vi "Indicators (SubVI).vi"(8 "read buffer":string) -> (9 "h5":dbl, 10 "zone 3":dbl, 11 "h6":dbl caption="h4", 12 "h1":dbl, 13 "h4":dbl, 14 "inlet air":dbl, 15 "h3":dbl, 16 "t1":dbl, 17 "h2":dbl, 18 "t2":dbl, 19 "t5":dbl, 20 "zone 1":dbl, 21 "t6":dbl, 22 "outlet":dbl, 23 "t3":dbl, 24 "zone 2":dbl, 25 "t4":dbl, 26 "main return":dbl)   [LabVIEW 2019]
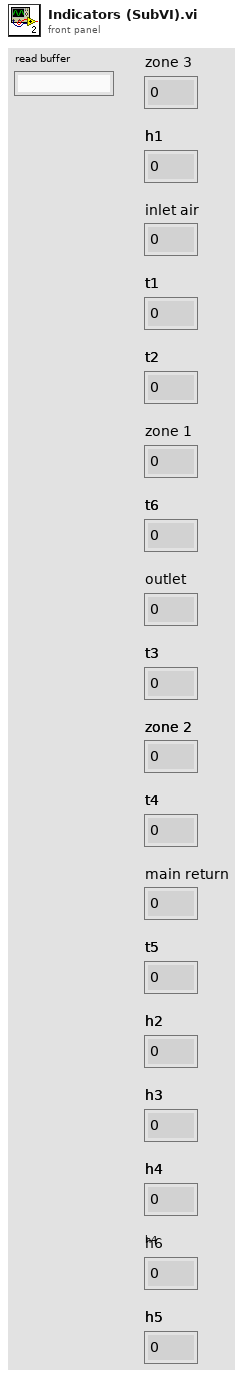
[diagram p1: front panel]
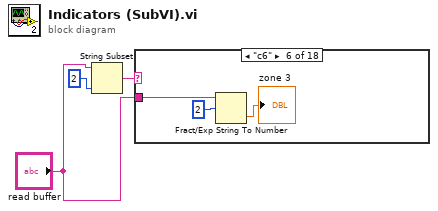
[diagram p0: block diagram]
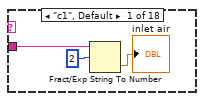
[diagram p2: hidden frame]
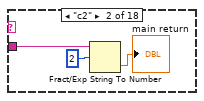
[diagram p3: hidden frame]
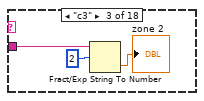
[diagram p4: hidden frame]
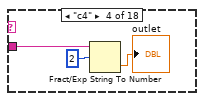
[diagram p5: hidden frame]
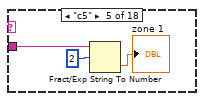
[diagram p6: hidden frame]
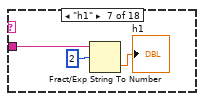
[diagram p7: hidden frame]
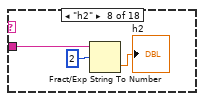
[diagram p8: hidden frame]
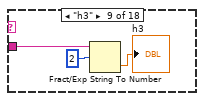
[diagram p9: hidden frame]
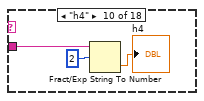
[diagram p10: hidden frame]
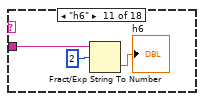
[diagram p11: hidden frame]
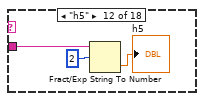
[diagram p12: hidden frame]
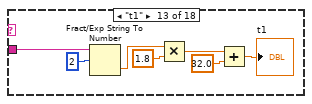
[diagram p13: hidden frame]
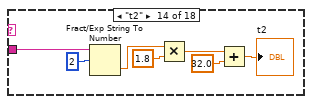
[diagram p14: hidden frame]
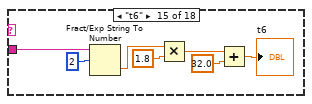
[diagram p15: hidden frame]
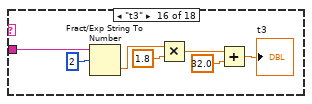
[diagram p16: hidden frame]
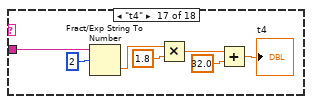
[diagram p17: hidden frame]
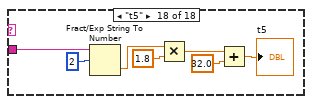
[diagram p18: hidden frame]
diagram:
  n1 = String Subset(string="read buffer", length (rest)=2 ("length (rest)")) -> (substring=w1:string)  [unwired: 1 in]
  n2 = case shown="\"c6\"" w1 {
    tunnel: "read buffer" -> [w5 w8 w11 w14 w17 w20 w23 w26 w29 w32 w35 w38 w45 w52 w59 w66 w73 w80]
    frame "c1", Default {
      n3 = Fract/Exp String To Number(string=w5, offset=2) -> (number=→"inlet air":dbl)  [unwired: 2 in, 1 out]
    }
    frame "c2" {
      n4 = Fract/Exp String To Number(string=w8, offset=2) -> (number=→"main return":dbl)  [unwired: 2 in, 1 out]
    }
    frame "c3" {
      n5 = Fract/Exp String To Number(string=w11, offset=2) -> (number=→"zone 2":dbl)  [unwired: 2 in, 1 out]
    }
    frame "c4" {
      n6 = Fract/Exp String To Number(string=w14, offset=2) -> (number=→"outlet":dbl)  [unwired: 2 in, 1 out]
    }
    frame "c5" {
      n7 = Fract/Exp String To Number(string=w17, offset=2) -> (number=→"zone 1":dbl)  [unwired: 2 in, 1 out]
    }
    frame "c6" {
      n8 = Fract/Exp String To Number(string=w20, offset=2) -> (number=→"zone 3":dbl)  [unwired: 2 in, 1 out]
    }
    frame "h1" {
      n9 = Fract/Exp String To Number(string=w23, offset=2) -> (number=→"h1":dbl)  [unwired: 2 in, 1 out]
    }
    frame "h2" {
      n10 = Fract/Exp String To Number(string=w26, offset=2) -> (number=→"h2":dbl)  [unwired: 2 in, 1 out]
    }
    frame "h3" {
      n11 = Fract/Exp String To Number(string=w29, offset=2) -> (number=→"h3":dbl)  [unwired: 2 in, 1 out]
    }
    frame "h4" {
      n12 = Fract/Exp String To Number(string=w32, offset=2) -> (number=→"h4":dbl)  [unwired: 2 in, 1 out]
    }
    frame "h6" {
      n13 = Fract/Exp String To Number(string=w35, offset=2) -> (number=→"h6":dbl)  [unwired: 2 in, 1 out]
    }
    frame "h5" {
      n14 = Fract/Exp String To Number(string=w38, offset=2) -> (number=→"h5":dbl)  [unwired: 2 in, 1 out]
    }
    frame "t1" {
      n15 = Fract/Exp String To Number(string=w45, offset=2) -> (number=w41:dbl)  [unwired: 2 in, 1 out]
      n16 = Multiply(x=w41, y=1.8) -> (x*y=w43:dbl)
      n17 = Add(x=w43, y=32.0) -> (x+y=→"t1":dbl)
    }
    frame "t2" {
      n18 = Fract/Exp String To Number(string=w52, offset=2) -> (number=w48:dbl)  [unwired: 2 in, 1 out]
      n19 = Multiply(x=w48, y=1.8) -> (x*y=w50:dbl)
      n20 = Add(x=w50, y=32.0) -> (x+y=→"t2":dbl)
    }
    frame "t6" {
      n21 = Fract/Exp String To Number(string=w59, offset=2) -> (number=w55:dbl)  [unwired: 2 in, 1 out]
      n22 = Multiply(x=w55, y=1.8) -> (x*y=w57:dbl)
      n23 = Add(x=w57, y=32.0) -> (x+y=→"t6":dbl)
    }
    frame "t3" {
      n24 = Fract/Exp String To Number(string=w66, offset=2) -> (number=w62:dbl)  [unwired: 2 in, 1 out]
      n25 = Multiply(x=w62, y=1.8) -> (x*y=w64:dbl)
      n26 = Add(x=w64, y=32.0) -> (x+y=→"t3":dbl)
    }
    frame "t4" {
      n27 = Fract/Exp String To Number(string=w73, offset=2) -> (number=w69:dbl)  [unwired: 2 in, 1 out]
      n28 = Multiply(x=w69, y=1.8) -> (x*y=w71:dbl)
      n29 = Add(x=w71, y=32.0) -> (x+y=→"t4":dbl)
    }
    frame "t5" {
      n30 = Fract/Exp String To Number(string=w80, offset=2) -> (number=w76:dbl)  [unwired: 2 in, 1 out]
      n31 = Multiply(x=w76, y=1.8) -> (x*y=w78:dbl)
      n32 = Add(x=w78, y=32.0) -> (x+y=→"t5":dbl)
    }
  }
